vi "initialise.vi"(8 "error in (no error)":errorcluster, 10 "points":dbl[][](array[numeric]), 11 "PointCollection in":refnum<class "PointCollection.lvclass">) -> (0 "error out":errorcluster, 3 "PointCollection out":refnum<class "PointCollection.lvclass">)   [LabVIEW 2010, in "PointCollection.lvclass"]
uses:
  PointCollection.lvclass
  PointCollection.lvclass/PointCollection.ctl
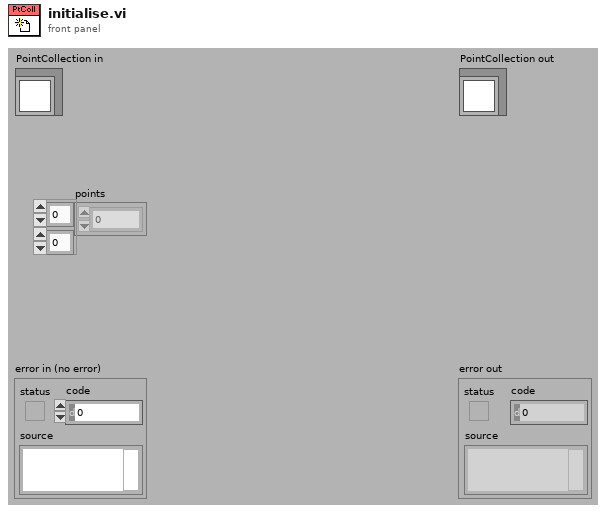
[diagram p1: front panel]
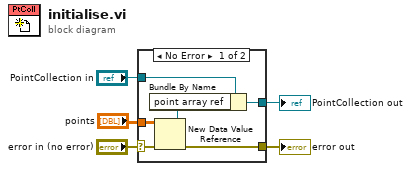
[diagram p0: block diagram]
diagram:
  n1 = case shown="No Error" "error in (no error)" {
    selector: "error in (no error)" -> [w9 w13]
    tunnel: [w6 w13] -> w4
    tunnel: [w10 w12] -> w2
    tunnel: "PointCollection in" -> [w11 w12]
    tunnel: "points" -> [w7 _]
    frame No Error {
      n2 = New Data Value Reference(data value=w7, error in=w9) -> (data value reference=w8:refnum<data-value>, error out=w6:errorcluster)
      n3 = Bundle By Name(cluster=w11, "point array ref"=w8) -> (w10:refnum<class "PointCollection.lvclass">)
    }
    frame Error {
    }
  }
  "error out" <- w4
  "PointCollection out" <- w2
